vi "LWXPS_ZygoPositionGet.vi"(8 "LabVIEW error IN":errorcluster, 11 "XPS Reference IN":refnum<k24>) -> (0 "XPS Error String":string, 1 "Position of Y axis":i64, 2 "Position of X axis":i64, 3 "Returned error code":i32, 4 "LabVIEW error OUT":errorcluster, 5 "XPS Reference OUT":refnum<k24>)   [LabVIEW 2014]
uses:
  D:/XPSQ8_LabView_Library/Development/Source/Dll/Newport.XPS.CommandInterface.dll
  Dll/Newport.XPS.CommandInterface.dll
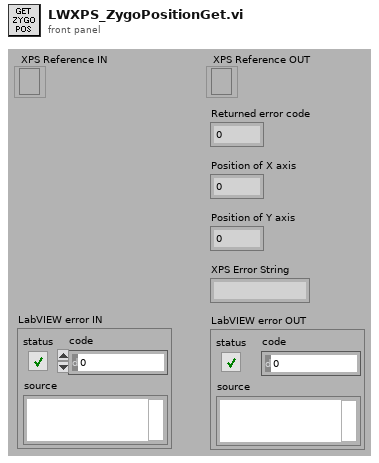
[diagram p1: front panel]
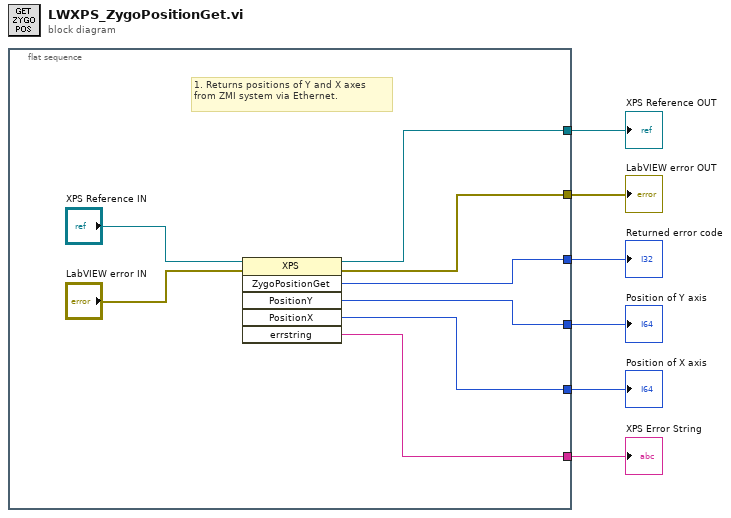
[diagram p0: block diagram]
diagram:
  n1 = flat-sequence {
    tunnel: [w12] -> w6
    tunnel: [w10] -> w5
    tunnel: [w13] -> w4
    tunnel: [w9] -> w1
    tunnel: [w8] -> w3
    tunnel: [w7] -> w2
    frame #0 {
      # "1. Returns positions of Y and X axes from ZMI system via Ethernet."
      n2 = invoke class="XPS" method="ZygoPositionGet"(reference="XPS Reference IN", error in="LabVIEW error IN") -> (reference out=w12:refnum<k24>, error out=w10:errorcluster, "ZygoPositionGet"=w13:i32, "PositionY"=w8:i64, "PositionX"=w9:i64, "errstring"=w7:string)  [unwired: 4 in]
    }
  }
  "XPS Error String" <- w2
  "XPS Reference OUT" <- w6
  "LabVIEW error OUT" <- w5
  "Returned error code" <- w4
  "Position of Y axis" <- w3
  "Position of X axis" <- w1
